vi "Autonomous Independent.vi"   [LabVIEW 2017]
doc: "This VI is called when autonomous begins, and will automatically be terminated when autonomous ends. You can carry out timed or sensor driven robot movement independently without needing to return to the caller."
uses:
  <vilib>/Rock Robotics/WPI/Utilities/WPI_GetSetVariantRefNum.vi
  <vilib>/Rock Robotics/Network Tables/NT Read String.vi
  <vilib>/Rock Robotics/Network Tables/NT Write Numeric Array.vi
  <vilib>/Rock Robotics/WPI/RobotDrive/WPI_RobotDriveArcadeDrive_Standard(NoSaturation).vi
panel:
  # "Be sure to right-click and choose Data Operations>>Make Current Value default if you want to save the array values with the VI"
types:
  T1 = typedef "WPI_JoystickDevRef.ctl" = cluster{"Device":T2}
  T2 = typedef "WPI_JoystickDeviceEnum.ctl" = enum16{"USB 0", "USB 1", "USB 2", "USB 3", "USB 4", "USB 5"}
  T3 = typedef "WPI_RobotDriveDevRef.ctl" = cluster{"DevStatus":errorcluster, "Motors[]":T4[], "Square Inputs":bool, "Max Output":dbl}
  T4 = typedef "WPI_MotorControlDeviceRef.ctl" = cluster{"DeviceStatus":errorcluster, "Type":T5, "PWM":cluster{"PWM Channel":T6, "DeadBand":T7}, "CAN":cluster{"Device Number":u8, "SetOutput VI Ref":variant, "GetOutput VI Ref":variant, "Enable VI Ref":variant, "Disable VI Ref":variant, "Data":variant}, "Invert":bool, "DIO PWM":cluster{"PWM \"Enable\" Channel":T6, "DIOChannel":T8, "PWM Rate":dbl}}
  T5 = typedef "WPI_MotorControlType.ctl" = enum16{"PWM", "CAN", "DIO PWM"}
  T6 = typedef "FPGA_DIOPWMChannel.ctl" = enum8{"PWM 0", "PWM 1", "PWM 2", "PWM 3", "PWM 4", "PWM 5", "PWM 6", "PWM 7", "PWM 8", "PWM 9", "PWM MXP 0", "PWM MXP 1", "PWM MXP 2", "PWM MXP 3", "PWM MXP 4", "PWM MXP 5", "PWM MXP 6", "PWM MXP 7", "PWM MXP 8", "PWM MXP 9", "Invalid"}
  T7 = typedef "WPI_PWMDeadband.ctl" = cluster{"Name":string, "maxPositivePwm":i32, "minPositivePwm":i32, "centerPwm":i32, "maxNegativePwm":i32, "minNegativePwm":i32, "angularRange":u16}
  T8 = typedef "FPGA_DIOChannel.ctl" = enum8{"DIO 0", "DIO 1", "DIO 2", "DIO 3", "DIO 4", "DIO 5", "DIO 6", "DIO 7", "DIO 8", "DIO 9", "DIO MXP 0", "DIO MXP 1", "DIO MXP 2", "DIO MXP 3", "DIO MXP 4", "DIO MXP 5", "DIO MXP 6", "DIO MXP 7", "DIO MXP 8", "DIO MXP 9", "DIO MXP 10", "DIO MXP 11", "DIO MXP 12", "DIO MXP 13", "DIO MXP 14", "DIO MXP 15", "SPI Port CS1", "SPI Port CS2", "SPI Port CS3", "SPI Port MISO", "SPI Port MOSI", "Invalid"}
  T9 = typedef "WPI_SwitchDevRef.ctl" = cluster{"DevStatus":errorcluster, "DIO Channel":T8, "CntIndex":T10, "Normally Closed":bool}
  T10 = typedef "FPGA_CounterCtrSystemIndex.ctl" = enum8{"Ctr 0", "Ctr 1", "Ctr 2", "Ctr 3", "Ctr 4", "Ctr 5", "Ctr 6", "Ctr 7", "Invalid"}
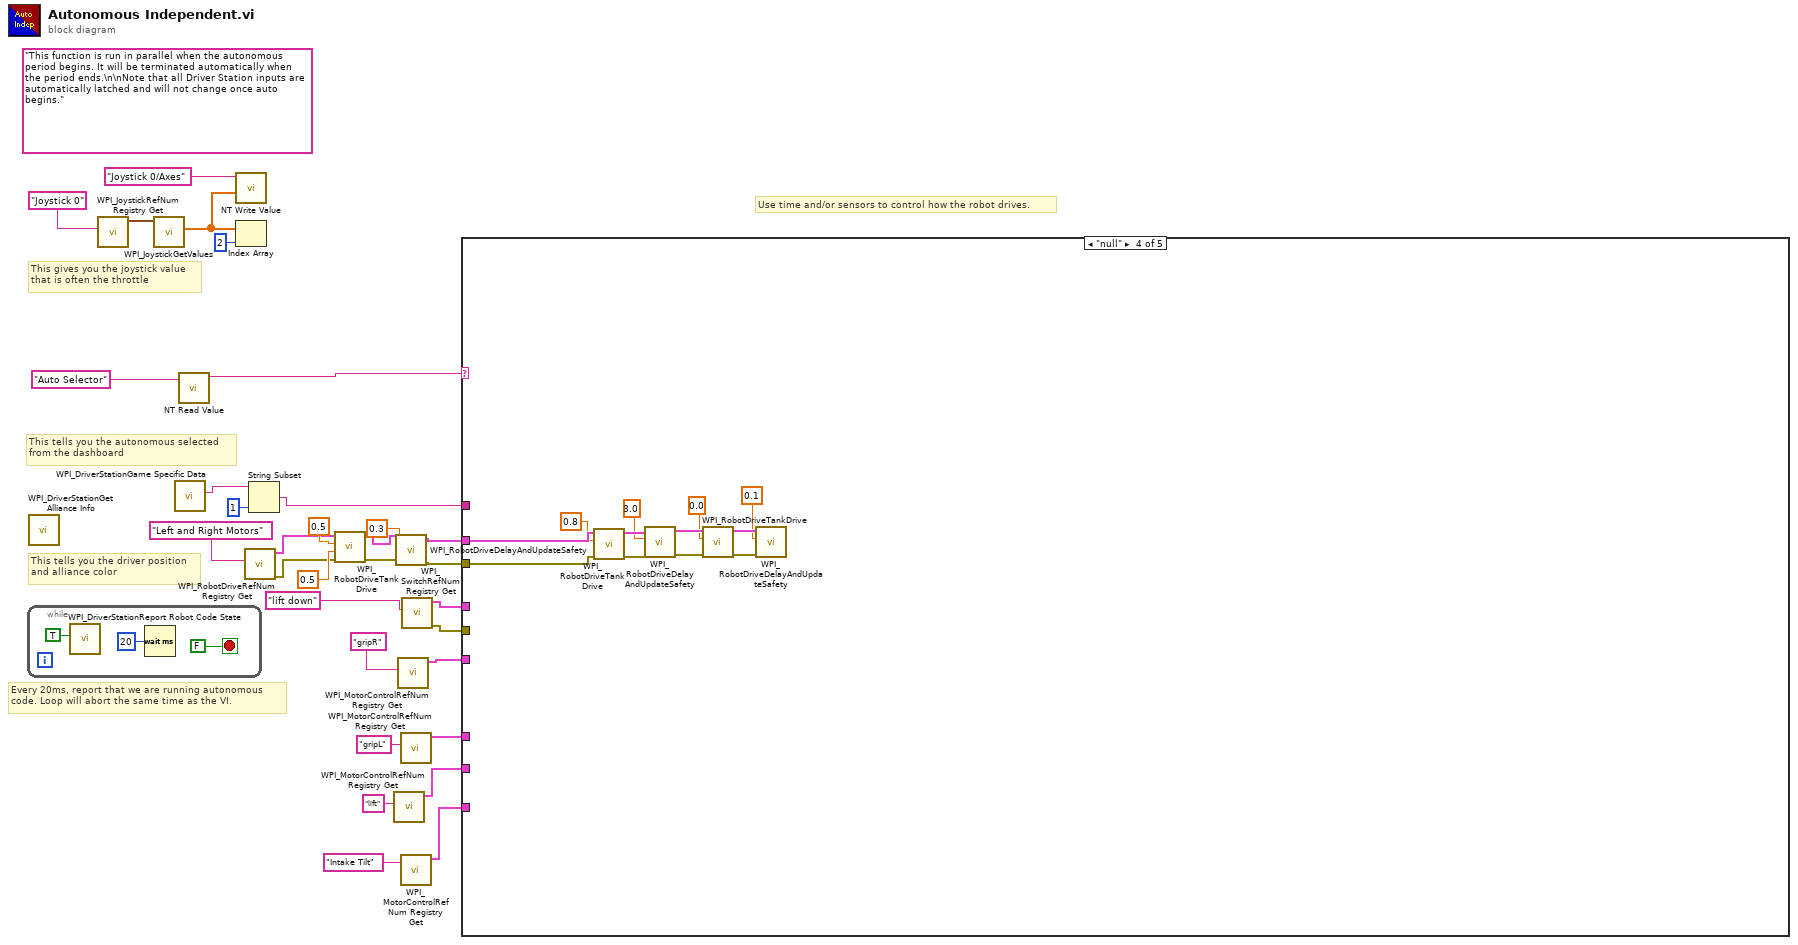
[diagram p0: block diagram]
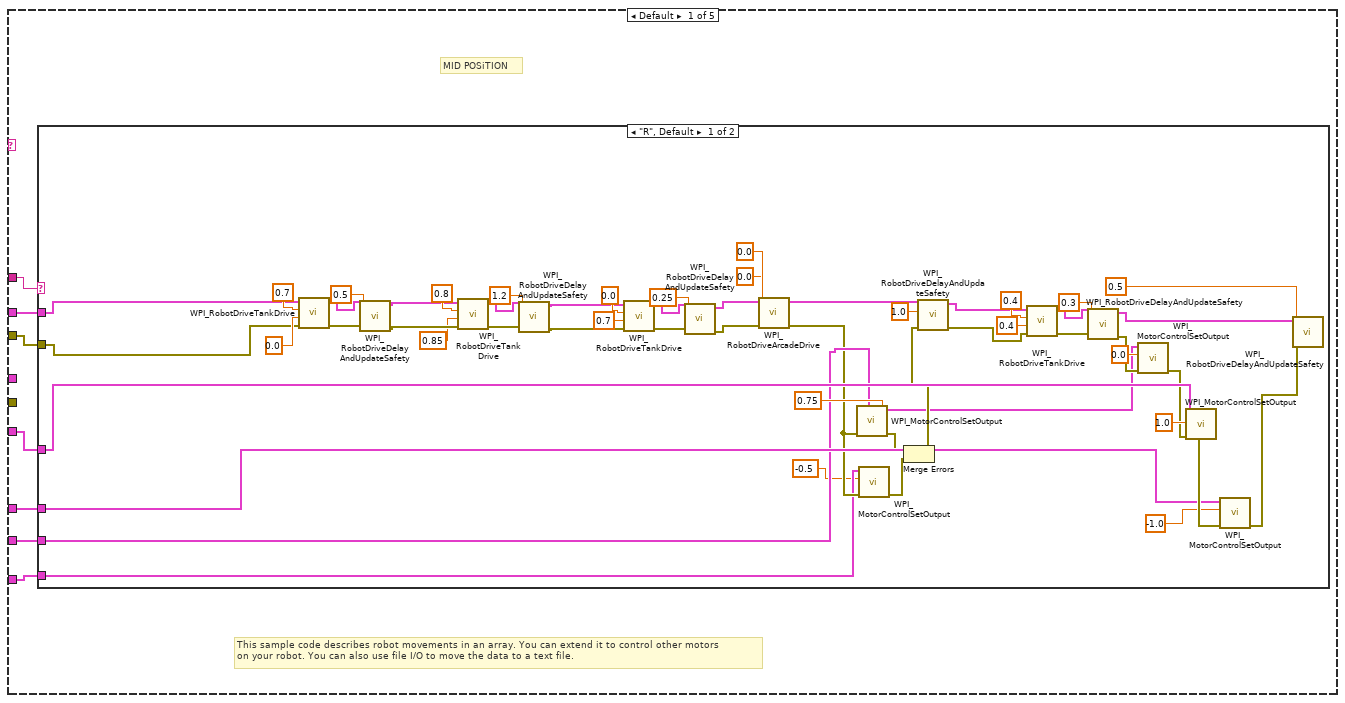
[diagram p2: hidden frame]
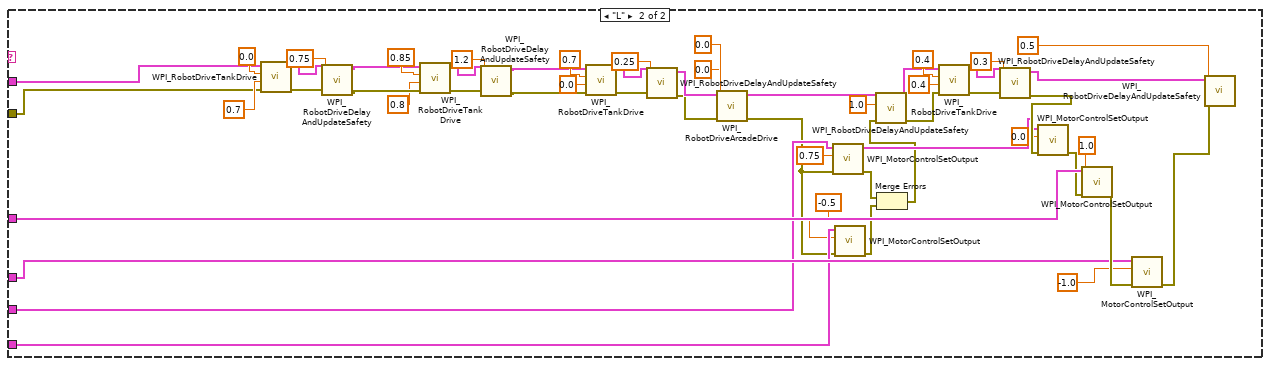
[diagram p3: hidden frame]
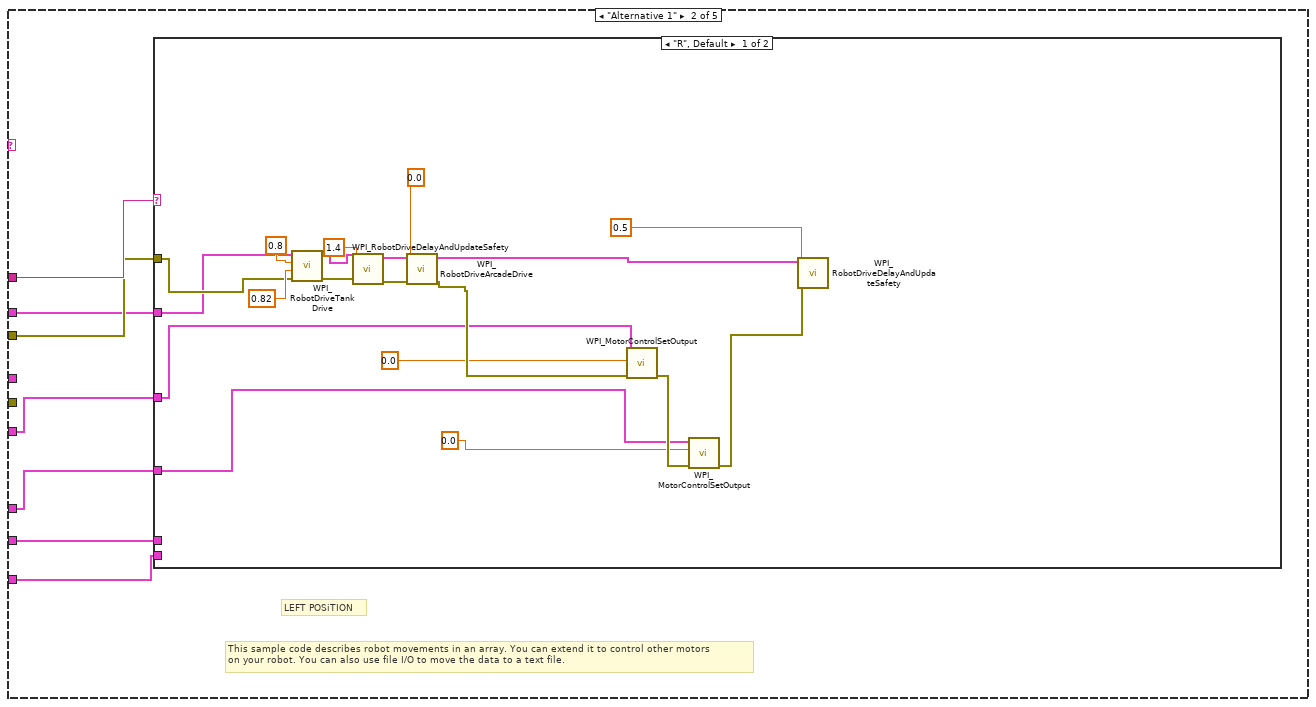
[diagram p4: hidden frame]
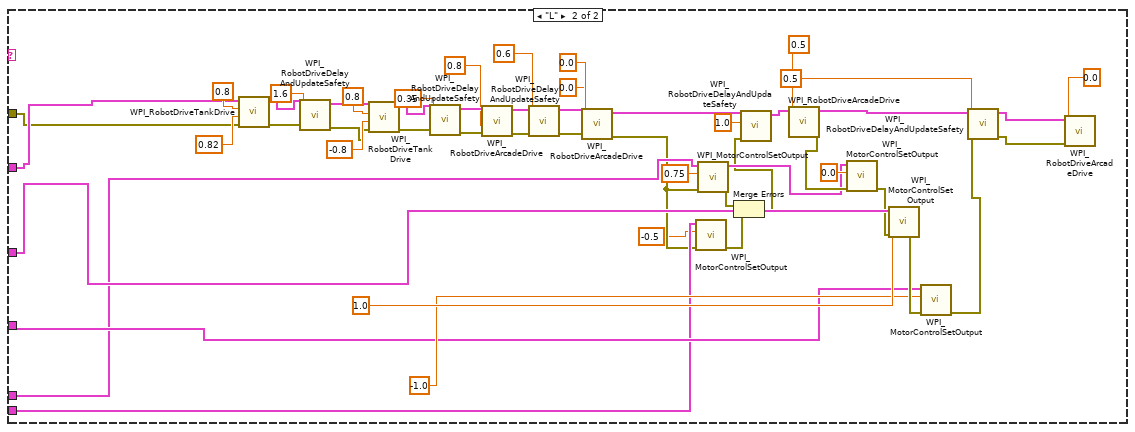
[diagram p5: hidden frame]
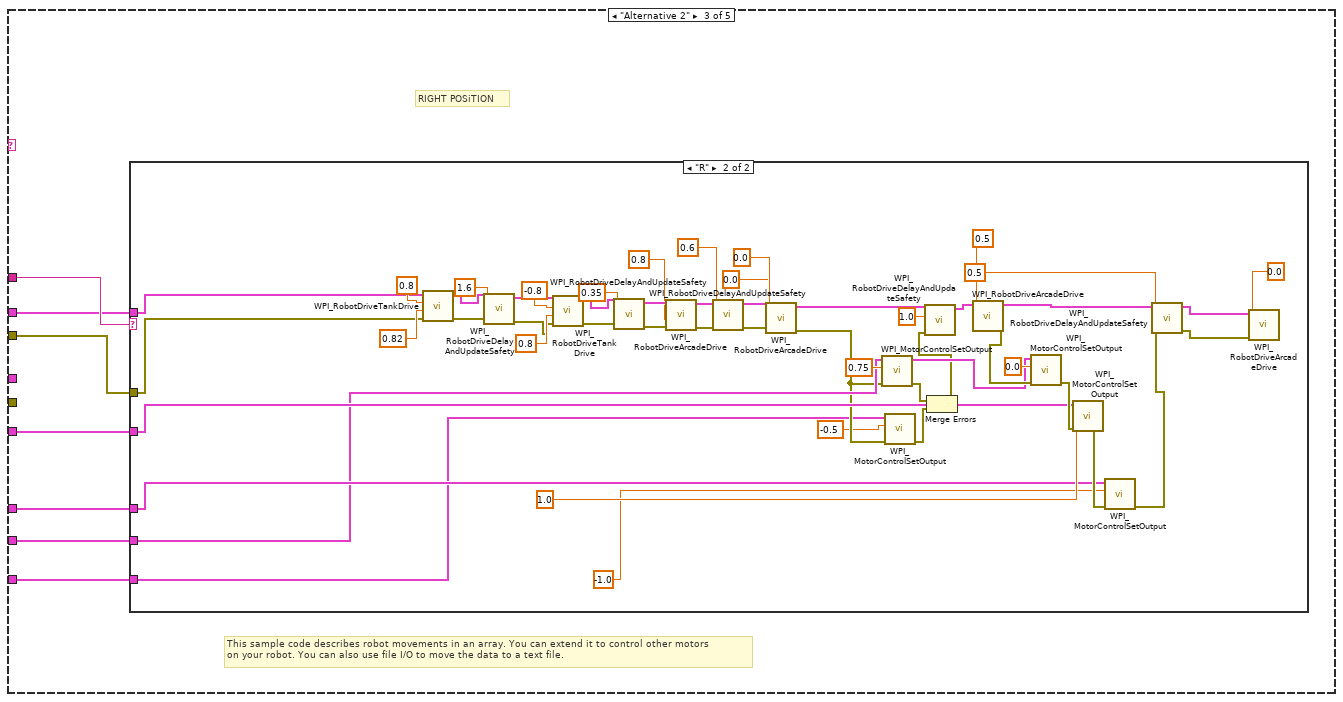
[diagram p6: hidden frame]
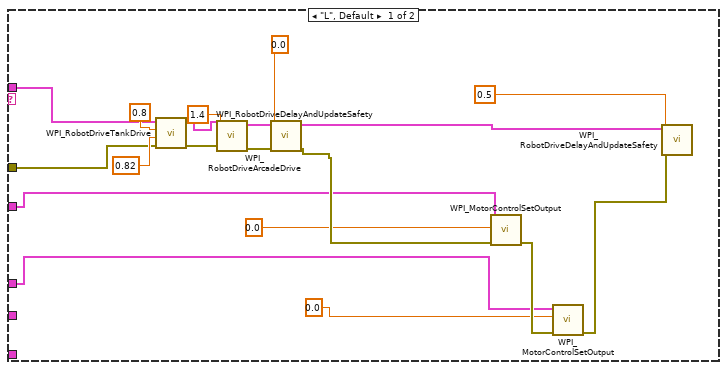
[diagram p7: hidden frame]
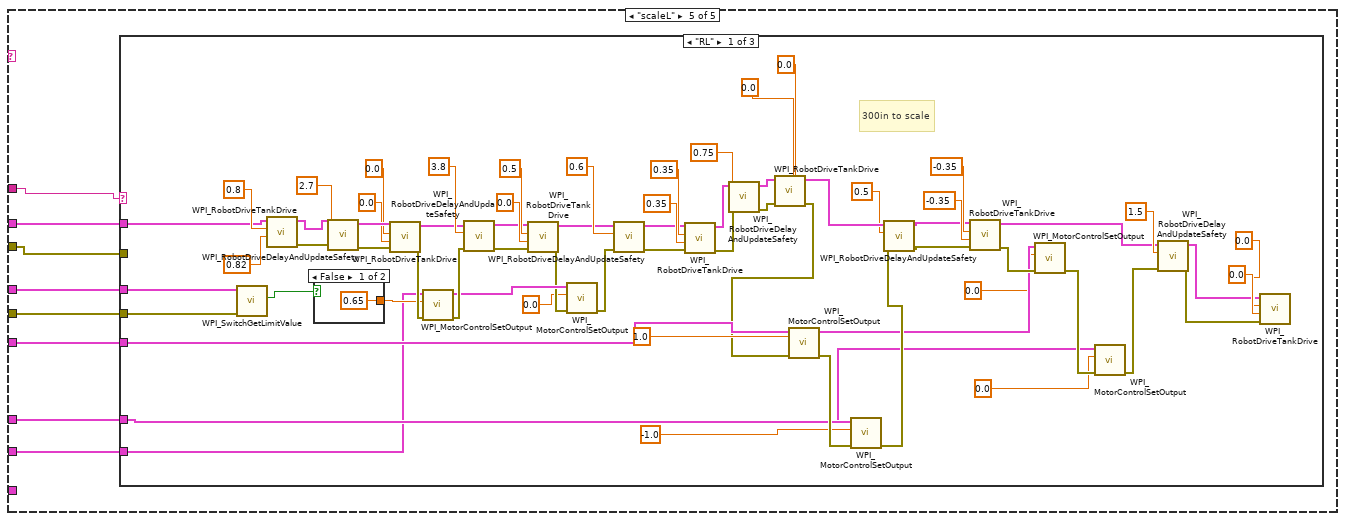
[diagram p8: hidden frame]
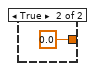
[diagram p9: hidden frame]
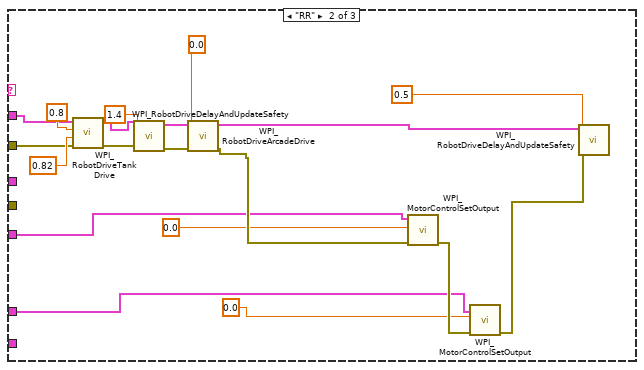
[diagram p10: hidden frame]
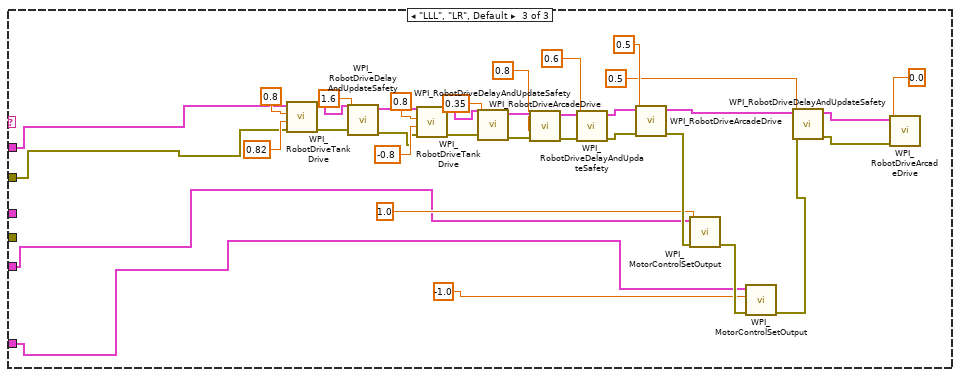
[diagram p11: hidden frame]
diagram:
  (unwired) "This function is run in parallel when the autonomous period begins. It will be terminated automatically when the period ends.\n\nNote that all Driver Station inputs are automatically latched and will not change once auto begins."
  # "This tells you the autonomous selected\nfrom the dashboard"
  # "Every 20ms, report that we are running autonomous\ncode. Loop will abort the same time as the VI."
  # "This gives you the joystick value\nthat is often the throttle"
  # "Use time and/or sensors to control how the robot drives."
  # "This tells you the driver position\nand alliance color"
  n1 = while {
    stop <- FALSE stop-if-true
    n2 = call <vilib>:"WPI_DriverStationReport Robot Code State.vi"("Autonomous"=TRUE) -> ()  [unwired: 10 in, 1 out]
    n3 = Wait (ms)(milliseconds to wait=u32 20) -> ()  [unwired: 1 out]
  }
  n4 = call <vilib>:"WPI_DriverStationGet Alliance Info.vi"() -> ()  [unwired: 12 out]
  n5 = call <vilib>:"WPI_JoystickRefNum Registry Get.vi"("refnum name"="Joystick 0") -> ("JoystickDevRef"=w30:T1)  [unwired: 1 in, 9 out]
  n6 = call <vilib>:"WPI_JoystickGetValues.vi"("JoystickDevRef"=w30) -> ("Axes"=w26:dbl[])  [unwired: 6 in, 4 out]
  n7 = call <vilib>:"WPI_DriverStationGame Specific Data.vi"() -> ("Game Specific Data"=w24:string)  [unwired: 11 in]
  n8 = call-poly <vilib>:"NT Read Value.vi"("Name"="Auto Selector") -> ("String"=w27:string)  [unwired: 9 in, 1 out]
  n9 = call-poly <vilib>:"NT Write Value.vi"("Numeric Array"=w26, "Name"="Joystick 0/Axes") -> ()  [unwired: 9 in, 1 out]
  n10 = Index Array(array=w26, index=2) -> ()  [unwired: 1 out]
  n11 = call <vilib>:"WPI_RobotDriveRefNum Registry Get.vi"("refnum name"="Left and Right Motors") -> ("error out"=w6:errorcluster, "RobotDriveDevRef"=w5:T3)  [unwired: 1 in, 8 out]
  n12 = String Subset(string=w24, length (rest)=1 ("length (rest)")) -> (substring=w22:string)  [unwired: 1 in]
  n13 = call <vilib>:"WPI_RobotDriveTankDrive.vi"("error in (no error)"=w6, "Right axis value"=0.5 ("Y axis value"), "Left axis value"=0.5 ("X axis value"), "RobotDriveDevRef"=w5) -> ("error out"=w10:errorcluster, "RobotDriveDevRef"=w9:T3)  [unwired: 5 in, 1 out]
  n14 = call <vilib>:"WPI_MotorControlRefNum Registry Get.vi"("refnum name"="lift") -> ("MotorControlDevRef"=w12:T4)  [unwired: 9 in, 1 out]
  n15 = call <vilib>:"WPI_RobotDriveDelayAndUpdateSafety.vi"("error in (no error)"=w10, "Delay (s)"=0.3, "RobotDriveDevRef"=w9) -> ("error out"=w3:errorcluster, "RobotDriveDevRef 2"=w4:T3)  [unwired: 7 in]
  n16 = call <vilib>:"WPI_MotorControlRefNum Registry Get.vi"("refnum name"="gripR") -> ("MotorControlDevRef"=w19:T4)  [unwired: 9 in, 1 out]
  n17 = call <vilib>:"WPI_MotorControlRefNum Registry Get.vi"("refnum name"="gripL") -> ("MotorControlDevRef"=w17:T4)  [unwired: 9 in, 1 out]
  n18 = call <vilib>:"WPI_MotorControlRefNum Registry Get.vi"("refnum name"="Intake Tilt") -> ("MotorControlDevRef"=w2:T4)  [unwired: 9 in, 1 out]
  n19 = call <vilib>:"WPI_SwitchRefNum Registry Get.vi"("refnum name"="lift down") -> ("error out"=w14:errorcluster, "SwitchDevRef"=w13:T9)  [unwired: 9 in]
  n20 = case shown="\"null\"" w27 {
    tunnel: w22 -> [w41 w156 w233 _ w323]
    tunnel: w3 -> [w40 w155 w232 w312 w316]
    tunnel: w19 -> [w39 w154 w231 _ w320]
    tunnel: w17 -> [w38 w153 w230 _ w321]
    tunnel: w4 -> [w37 w152 w229 w313 w322]
    tunnel: w14 -> [_ _ _ _ w319]
    tunnel: w13 -> [_ _ _ _ w318]
    tunnel: w12 -> [w36 w151 w228 _ w317]
    tunnel: w2 -> [w35 w150 w227 _ _]
    frame Default {
      # "MID POSiTION"
      # "This sample code describes robot movements in an array. You can extend it to control other motors\non your robot. You can also use file I/O to move the data to a text file."
      n21 = case shown="\"R\", Default" w41 {
        tunnel: w40 -> [w85 w119]
        tunnel: w39 -> [w84 w118]
        tunnel: w38 -> [w83 w117]
        tunnel: w37 -> [w62 w116]
        tunnel: w36 -> [w52 w106]
        tunnel: w35 -> [w44 w101]
        frame "R", Default {
          n22 = call <vilib>:"WPI_RobotDriveTankDrive.vi"("error in (no error)"=w85, "Right axis value"=0.0 ("Y axis value"), "Left axis value"=0.7 ("X axis value"), "RobotDriveDevRef"=w62) -> ("error out"=w91:errorcluster, "RobotDriveDevRef"=w90:T3)  [unwired: 5 in, 1 out]
          n23 = call <vilib>:"WPI_RobotDriveDelayAndUpdateSafety.vi"("error in (no error)"=w91, "Delay (s)"=0.5, "RobotDriveDevRef"=w90) -> ("error out"=w77:errorcluster, "RobotDriveDevRef 2"=w78:T3)  [unwired: 7 in]
          n24 = call <vilib>:"WPI_RobotDriveTankDrive.vi"("error in (no error)"=w77, "Right axis value"=0.85, "Left axis value"=0.8 ("X axis value"), "RobotDriveDevRef"=w78) -> ("error out"=w81:errorcluster, "RobotDriveDevRef"=w80:T3)  [unwired: 5 in, 1 out]
          n25 = call <vilib>:"WPI_RobotDriveDelayAndUpdateSafety.vi"("error in (no error)"=w81, "Delay (s)"=1.2, "RobotDriveDevRef"=w80) -> ("error out"=w70:errorcluster, "RobotDriveDevRef 2"=w71:T3)  [unwired: 7 in]
          n26 = call <vilib>:"WPI_RobotDriveTankDrive.vi"("error in (no error)"=w70, "Right axis value"=0.7, "Left axis value"=0.0 ("X axis value"), "RobotDriveDevRef"=w71) -> ("error out"=w74:errorcluster, "RobotDriveDevRef"=w73:T3)  [unwired: 5 in, 1 out]
          n27 = call <vilib>:"WPI_RobotDriveDelayAndUpdateSafety.vi"("error in (no error)"=w74, "Delay (s)"=0.25, "RobotDriveDevRef"=w73) -> ("error out"=w55:errorcluster, "RobotDriveDevRef 2"=w56:T3)  [unwired: 7 in]
          n28 = call-poly <vilib>:"WPI_RobotDriveArcadeDrive.vi"("error in (no error)"=w55, "Y axis value"=0.0, "X axis value"=0.0, "RobotDriveDevRef"=w56) -> ("error out"=w48:errorcluster, "RobotDriveDevRef"=w61:T3)  [unwired: 5 in, 1 out]
          n29 = call <vilib>:"WPI_MotorControlSetOutput.vi"("error in (no error)"=w48, "Output"=0.75, "MotorControlDevRef"=w52) -> ("error out"=w47:errorcluster, "MotorControlDevRef"=w42:T4)  [unwired: 6 in, 1 out]
          n30 = call <vilib>:"WPI_MotorControlSetOutput.vi"("error in (no error)"=w48, "Output"=-0.5, "MotorControlDevRef"=w44) -> ("error out"=w46:errorcluster)  [unwired: 6 in, 2 out]
          n31 = Merge Errors(w47, w46) -> (w45:errorcluster)
          n32 = call <vilib>:"WPI_RobotDriveDelayAndUpdateSafety.vi"("error in (no error)"=w45, "Delay (s)"=1.0, "RobotDriveDevRef"=w61) -> ("error out"=w53:errorcluster, "RobotDriveDevRef 2"=w54:T3)  [unwired: 7 in]
          n33 = call <vilib>:"WPI_RobotDriveTankDrive.vi"("error in (no error)"=w53, "Right axis value"=0.4, "Left axis value"=0.4 ("X axis value"), "RobotDriveDevRef"=w54) -> ("error out"=w67:errorcluster, "RobotDriveDevRef"=w66:T3)  [unwired: 5 in, 1 out]
          n34 = call <vilib>:"WPI_RobotDriveDelayAndUpdateSafety.vi"("error in (no error)"=w67, "Delay (s)"=0.3, "RobotDriveDevRef"=w66) -> ("error out"=w51:errorcluster, "RobotDriveDevRef 2"=w63:T3)  [unwired: 7 in]
          n35 = call <vilib>:"WPI_MotorControlSetOutput.vi"("error in (no error)"=w51, "Output"=0.0, "MotorControlDevRef"=w42) -> ("error out"=w50:errorcluster)  [unwired: 6 in, 2 out]
          n36 = call <vilib>:"WPI_MotorControlSetOutput.vi"("error in (no error)"=w50, "Output"=1.0, "MotorControlDevRef"=w84) -> ("error out"=w93:errorcluster)  [unwired: 6 in, 2 out]
          n37 = call <vilib>:"WPI_MotorControlSetOutput.vi"("error in (no error)"=w93, "Output"=-1.0, "MotorControlDevRef"=w83) -> ("error out"=w92:errorcluster)  [unwired: 6 in, 2 out]
          n38 = call <vilib>:"WPI_RobotDriveDelayAndUpdateSafety.vi"("error in (no error)"=w92, "Delay (s)"=0.5, "RobotDriveDevRef"=w63) -> ()  [unwired: 7 in, 2 out]
        }
        frame "L" {
          n39 = call <vilib>:"WPI_RobotDriveTankDrive.vi"("error in (no error)"=w119, "Right axis value"=0.7 ("Y axis value"), "Left axis value"=0.0 ("X axis value"), "RobotDriveDevRef"=w116) -> ("error out"=w145:errorcluster, "RobotDriveDevRef"=w144:T3)  [unwired: 5 in, 1 out]
          n40 = call <vilib>:"WPI_RobotDriveDelayAndUpdateSafety.vi"("error in (no error)"=w145, "Delay (s)"=0.75, "RobotDriveDevRef"=w144) -> ("error out"=w134:errorcluster, "RobotDriveDevRef 2"=w135:T3)  [unwired: 7 in]
          n41 = call <vilib>:"WPI_RobotDriveTankDrive.vi"("error in (no error)"=w134, "Right axis value"=0.8, "Left axis value"=0.85 ("X axis value"), "RobotDriveDevRef"=w135) -> ("error out"=w138:errorcluster, "RobotDriveDevRef"=w137:T3)  [unwired: 5 in, 1 out]
          n42 = call <vilib>:"WPI_RobotDriveDelayAndUpdateSafety.vi"("error in (no error)"=w138, "Delay (s)"=1.2, "RobotDriveDevRef"=w137) -> ("error out"=w127:errorcluster, "RobotDriveDevRef 2"=w128:T3)  [unwired: 7 in]
          n43 = call <vilib>:"WPI_RobotDriveTankDrive.vi"("error in (no error)"=w127, "Right axis value"=0.0, "Left axis value"=0.7 ("X axis value"), "RobotDriveDevRef"=w128) -> ("error out"=w131:errorcluster, "RobotDriveDevRef"=w130:T3)  [unwired: 5 in, 1 out]
          n44 = call <vilib>:"WPI_RobotDriveDelayAndUpdateSafety.vi"("error in (no error)"=w131, "Delay (s)"=0.25, "RobotDriveDevRef"=w130) -> ("error out"=w109:errorcluster, "RobotDriveDevRef 2"=w110:T3)  [unwired: 7 in]
          n45 = call-poly <vilib>:"WPI_RobotDriveArcadeDrive.vi"("error in (no error)"=w109, "Y axis value"=0.0, "X axis value"=0.0, "RobotDriveDevRef"=w110) -> ("error out"=w100:errorcluster, "RobotDriveDevRef"=w115:T3)  [unwired: 5 in, 1 out]
          n46 = call <vilib>:"WPI_MotorControlSetOutput.vi"("error in (no error)"=w100, "Output"=0.75, "MotorControlDevRef"=w106) -> ("error out"=w99:errorcluster, "MotorControlDevRef"=w103:T4)  [unwired: 6 in, 1 out]
          n47 = call <vilib>:"WPI_MotorControlSetOutput.vi"("error in (no error)"=w100, "Output"=-0.5, "MotorControlDevRef"=w101) -> ("error out"=w98:errorcluster)  [unwired: 6 in, 2 out]
          n48 = Merge Errors(w99, w98) -> (w97:errorcluster)
          n49 = call <vilib>:"WPI_RobotDriveDelayAndUpdateSafety.vi"("error in (no error)"=w97, "Delay (s)"=1.0, "RobotDriveDevRef"=w115) -> ("error out"=w107:errorcluster, "RobotDriveDevRef 2"=w108:T3)  [unwired: 7 in]
          n50 = call <vilib>:"WPI_RobotDriveTankDrive.vi"("error in (no error)"=w107, "Right axis value"=0.4, "Left axis value"=0.4 ("X axis value"), "RobotDriveDevRef"=w108) -> ("error out"=w124:errorcluster, "RobotDriveDevRef"=w123:T3)  [unwired: 5 in, 1 out]
          n51 = call <vilib>:"WPI_RobotDriveDelayAndUpdateSafety.vi"("error in (no error)"=w124, "Delay (s)"=0.3, "RobotDriveDevRef"=w123) -> ("error out"=w105:errorcluster, "RobotDriveDevRef 2"=w120:T3)  [unwired: 7 in]
          n52 = call <vilib>:"WPI_MotorControlSetOutput.vi"("error in (no error)"=w105, "Output"=0.0, "MotorControlDevRef"=w103) -> ("error out"=w104:errorcluster)  [unwired: 6 in, 2 out]
          n53 = call <vilib>:"WPI_MotorControlSetOutput.vi"("error in (no error)"=w104, "Output"=1.0, "MotorControlDevRef"=w118) -> ("error out"=w147:errorcluster)  [unwired: 6 in, 2 out]
          n54 = call <vilib>:"WPI_MotorControlSetOutput.vi"("error in (no error)"=w147, "Output"=-1.0, "MotorControlDevRef"=w117) -> ("error out"=w146:errorcluster)  [unwired: 6 in, 2 out]
          n55 = call <vilib>:"WPI_RobotDriveDelayAndUpdateSafety.vi"("error in (no error)"=w146, "Delay (s)"=0.5, "RobotDriveDevRef"=w120) -> ()  [unwired: 7 in, 2 out]
        }
      }
    }
    frame "Alternative 1" {
      # "LEFT POSiTION"
      # "This sample code describes robot movements in an array. You can extend it to control other motors\non your robot. You can also use file I/O to move the data to a text file."
      n56 = case shown="\"R\", Default" w156 {
        tunnel: w155 -> [w160 w206]
        tunnel: w154 -> [w159 w205]
        tunnel: w153 -> [w158 w204]
        tunnel: w152 -> [w157 w207]
        tunnel: w151 -> [_ w186]
        tunnel: w150 -> [_ w181]
        frame "R", Default {
          n57 = call <vilib>:"WPI_RobotDriveTankDrive.vi"("error in (no error)"=w160, "Right axis value"=0.82 ("Y axis value"), "Left axis value"=0.8 ("X axis value"), "RobotDriveDevRef"=w157) -> ("error out"=w166:errorcluster, "RobotDriveDevRef"=w165:T3)  [unwired: 5 in, 1 out]
          n58 = call <vilib>:"WPI_RobotDriveDelayAndUpdateSafety.vi"("error in (no error)"=w166, "Delay (s)"=1.4, "RobotDriveDevRef"=w165) -> ("error out"=w174:errorcluster, "RobotDriveDevRef 2"=w173:T3)  [unwired: 7 in]
          n59 = call-poly <vilib>:"WPI_RobotDriveArcadeDrive.vi"("error in (no error)"=w174, "Y axis value"=0.0, "RobotDriveDevRef"=w173) -> ("error out"=w168:errorcluster, "RobotDriveDevRef"=w171:T3)  [unwired: 6 in, 1 out]
          n60 = call <vilib>:"WPI_MotorControlSetOutput.vi"("error in (no error)"=w168, "Output"=0.0, "MotorControlDevRef"=w159) -> ("error out"=w169:errorcluster)  [unwired: 6 in, 2 out]
          n61 = call <vilib>:"WPI_MotorControlSetOutput.vi"("error in (no error)"=w169, "Output"=0.0, "MotorControlDevRef"=w158) -> ("error out"=w167:errorcluster)  [unwired: 6 in, 2 out]
          n62 = call <vilib>:"WPI_RobotDriveDelayAndUpdateSafety.vi"("error in (no error)"=w167, "Delay (s)"=0.5, "RobotDriveDevRef"=w171) -> ()  [unwired: 7 in, 2 out]
        }
        frame "L" {
          n63 = call <vilib>:"WPI_RobotDriveTankDrive.vi"("error in (no error)"=w206, "Right axis value"=0.82 ("Y axis value"), "Left axis value"=0.8 ("X axis value"), "RobotDriveDevRef"=w207) -> ("error out"=w220:errorcluster, "RobotDriveDevRef"=w219:T3)  [unwired: 5 in, 1 out]
          n64 = call <vilib>:"WPI_RobotDriveDelayAndUpdateSafety.vi"("error in (no error)"=w220, "Delay (s)"=1.6, "RobotDriveDevRef"=w219) -> ("error out"=w208:errorcluster, "RobotDriveDevRef 2"=w209:T3)  [unwired: 7 in]
          n65 = call <vilib>:"WPI_RobotDriveTankDrive.vi"("error in (no error)"=w208, "Right axis value"=-0.8 ("Y axis value"), "Left axis value"=0.8 ("X axis value"), "RobotDriveDevRef"=w209) -> ("error out"=w213:errorcluster, "RobotDriveDevRef"=w212:T3)  [unwired: 5 in, 1 out]
          n66 = call <vilib>:"WPI_RobotDriveDelayAndUpdateSafety.vi"("error in (no error)"=w213, "Delay (s)"=0.35, "RobotDriveDevRef"=w212) -> ("error out"=w199:errorcluster, "RobotDriveDevRef 2"=w200:T3)  [unwired: 7 in]
          n67 = call-poly <vilib>:"WPI_RobotDriveArcadeDrive.vi"("error in (no error)"=w199, "Y axis value"=0.8, "RobotDriveDevRef"=w200) -> ("error out"=w196:errorcluster, "RobotDriveDevRef"=w197:T3)  [unwired: 6 in, 1 out]
          n68 = call <vilib>:"WPI_RobotDriveDelayAndUpdateSafety.vi"("error in (no error)"=w196, "Delay (s)"=0.6, "RobotDriveDevRef"=w197) -> ("error out"=w194:errorcluster, "RobotDriveDevRef 2"=w193:T3)  [unwired: 7 in]
          n69 = call-poly <vilib>:"WPI_RobotDriveArcadeDrive.vi"("error in (no error)"=w194, "Y axis value"=0.0, "X axis value"=0.0, "RobotDriveDevRef"=w193) -> ("error out"=w180:errorcluster, "RobotDriveDevRef"=w192:T3)  [unwired: 5 in, 1 out]
          n70 = call <vilib>:"WPI_MotorControlSetOutput.vi"("error in (no error)"=w180, "Output"=-0.5, "MotorControlDevRef"=w181) -> ("error out"=w178:errorcluster)  [unwired: 6 in, 2 out]
          n71 = call <vilib>:"WPI_MotorControlSetOutput.vi"("error in (no error)"=w180, "Output"=0.75, "MotorControlDevRef"=w186) -> ("error out"=w179:errorcluster, "MotorControlDevRef"=w182:T4)  [unwired: 6 in, 1 out]
          n72 = Merge Errors(w179, w178) -> (w177:errorcluster)
          n73 = call <vilib>:"WPI_RobotDriveDelayAndUpdateSafety.vi"("error in (no error)"=w177, "Delay (s)"=1.0, "RobotDriveDevRef"=w192) -> ("RobotDriveDevRef 2"=w191:T3)  [unwired: 7 in, 1 out]
          n74 = call-poly <vilib>:"WPI_RobotDriveArcadeDrive.vi"("Y axis value"=0.5, "RobotDriveDevRef"=w191) -> ("error out"=w184:errorcluster, "RobotDriveDevRef"=w224:T3)  [unwired: 7 in, 1 out]
          n75 = call <vilib>:"WPI_MotorControlSetOutput.vi"("error in (no error)"=w184, "Output"=0.0, "MotorControlDevRef"=w182) -> ("error out"=w183:errorcluster)  [unwired: 6 in, 2 out]
          n76 = call <vilib>:"WPI_MotorControlSetOutput.vi"("error in (no error)"=w183, "Output"=1.0, "MotorControlDevRef"=w205) -> ("error out"=w222:errorcluster)  [unwired: 6 in, 2 out]
          n77 = call <vilib>:"WPI_MotorControlSetOutput.vi"("error in (no error)"=w222, "Output"=-1.0, "MotorControlDevRef"=w204) -> ("error out"=w221:errorcluster)  [unwired: 6 in, 2 out]
          n78 = call <vilib>:"WPI_RobotDriveDelayAndUpdateSafety.vi"("error in (no error)"=w221, "Delay (s)"=0.5, "RobotDriveDevRef"=w224) -> ("error out"=w201:errorcluster, "RobotDriveDevRef 2"=w202:T3)  [unwired: 7 in]
          n79 = call-poly <vilib>:"WPI_RobotDriveArcadeDrive.vi"("error in (no error)"=w201, "Y axis value"=0.0, "RobotDriveDevRef"=w202) -> ()  [unwired: 6 in, 3 out]
        }
      }
    }
    frame "Alternative 2" {
      # "RIGHT POSiTION"
      # "This sample code describes robot movements in an array. You can extend it to control other motors\non your robot. You can also use file I/O to move the data to a text file."
      n80 = case shown="\"R\"" w233 {
        tunnel: w232 -> [w235 w262]
        tunnel: w231 -> [w236 w261]
        tunnel: w230 -> [w237 w260]
        tunnel: w229 -> [w234 w263]
        tunnel: w228 -> [_ w259]
        tunnel: w227 -> [_ w257]
        frame "L", Default {
          n81 = call <vilib>:"WPI_RobotDriveTankDrive.vi"("error in (no error)"=w235, "Right axis value"=0.82 ("Y axis value"), "Left axis value"=0.8 ("X axis value"), "RobotDriveDevRef"=w234) -> ("error out"=w243:errorcluster, "RobotDriveDevRef"=w242:T3)  [unwired: 5 in, 1 out]
          n82 = call <vilib>:"WPI_RobotDriveDelayAndUpdateSafety.vi"("error in (no error)"=w243, "Delay (s)"=1.4, "RobotDriveDevRef"=w242) -> ("error out"=w251:errorcluster, "RobotDriveDevRef 2"=w250:T3)  [unwired: 7 in]
          n83 = call-poly <vilib>:"WPI_RobotDriveArcadeDrive.vi"("error in (no error)"=w251, "Y axis value"=0.0, "RobotDriveDevRef"=w250) -> ("error out"=w245:errorcluster, "RobotDriveDevRef"=w248:T3)  [unwired: 6 in, 1 out]
          n84 = call <vilib>:"WPI_MotorControlSetOutput.vi"("error in (no error)"=w245, "Output"=0.0, "MotorControlDevRef"=w236) -> ("error out"=w246:errorcluster)  [unwired: 6 in, 2 out]
          n85 = call <vilib>:"WPI_MotorControlSetOutput.vi"("error in (no error)"=w246, "Output"=0.0, "MotorControlDevRef"=w237) -> ("error out"=w244:errorcluster)  [unwired: 6 in, 2 out]
          n86 = call <vilib>:"WPI_RobotDriveDelayAndUpdateSafety.vi"("error in (no error)"=w244, "Delay (s)"=0.5, "RobotDriveDevRef"=w248) -> ()  [unwired: 7 in, 2 out]
        }
        frame "R" {
          n87 = call <vilib>:"WPI_RobotDriveTankDrive.vi"("error in (no error)"=w262, "Right axis value"=0.82 ("Y axis value"), "Left axis value"=0.8 ("X axis value"), "RobotDriveDevRef"=w263) -> ("error out"=w297:errorcluster, "RobotDriveDevRef"=w296:T3)  [unwired: 5 in, 1 out]
          n88 = call <vilib>:"WPI_RobotDriveDelayAndUpdateSafety.vi"("error in (no error)"=w297, "Delay (s)"=1.6, "RobotDriveDevRef"=w296) -> ("error out"=w285:errorcluster, "RobotDriveDevRef 2"=w286:T3)  [unwired: 7 in]
          n89 = call <vilib>:"WPI_RobotDriveTankDrive.vi"("error in (no error)"=w285, "Right axis value"=0.8 ("Y axis value"), "Left axis value"=-0.8 ("X axis value"), "RobotDriveDevRef"=w286) -> ("error out"=w290:errorcluster, "RobotDriveDevRef"=w289:T3)  [unwired: 5 in, 1 out]
          n90 = call <vilib>:"WPI_RobotDriveDelayAndUpdateSafety.vi"("error in (no error)"=w290, "Delay (s)"=0.35, "RobotDriveDevRef"=w289) -> ("error out"=w280:errorcluster, "RobotDriveDevRef 2"=w281:T3)  [unwired: 7 in]
          n91 = call-poly <vilib>:"WPI_RobotDriveArcadeDrive.vi"("error in (no error)"=w280, "Y axis value"=0.8, "RobotDriveDevRef"=w281) -> ("error out"=w277:errorcluster, "RobotDriveDevRef"=w278:T3)  [unwired: 6 in, 1 out]
          n92 = call <vilib>:"WPI_RobotDriveDelayAndUpdateSafety.vi"("error in (no error)"=w277, "Delay (s)"=0.6, "RobotDriveDevRef"=w278) -> ("error out"=w275:errorcluster, "RobotDriveDevRef 2"=w274:T3)  [unwired: 7 in]
          n93 = call-poly <vilib>:"WPI_RobotDriveArcadeDrive.vi"("error in (no error)"=w275, "Y axis value"=0.0, "X axis value"=0.0, "RobotDriveDevRef"=w274) -> ("error out"=w258:errorcluster, "RobotDriveDevRef"=w273:T3)  [unwired: 5 in, 1 out]
          n94 = call <vilib>:"WPI_MotorControlSetOutput.vi"("error in (no error)"=w258, "Output"=0.75, "MotorControlDevRef"=w259) -> ("error out"=w256:errorcluster, "MotorControlDevRef"=w264:T4)  [unwired: 6 in, 1 out]
          n95 = call <vilib>:"WPI_MotorControlSetOutput.vi"("error in (no error)"=w258, "Output"=-0.5, "MotorControlDevRef"=w257) -> ("error out"=w255:errorcluster)  [unwired: 6 in, 2 out]
          n96 = Merge Errors(w256, w255) -> (w254:errorcluster)
          n97 = call <vilib>:"WPI_RobotDriveDelayAndUpdateSafety.vi"("error in (no error)"=w254, "Delay (s)"=1.0, "RobotDriveDevRef"=w273) -> ("RobotDriveDevRef 2"=w272:T3)  [unwired: 7 in, 1 out]
          n98 = call-poly <vilib>:"WPI_RobotDriveArcadeDrive.vi"("Y axis value"=0.5, "RobotDriveDevRef"=w272) -> ("error out"=w266:errorcluster, "RobotDriveDevRef"=w301:T3)  [unwired: 7 in, 1 out]
          n99 = call <vilib>:"WPI_MotorControlSetOutput.vi"("error in (no error)"=w266, "Output"=0.0, "MotorControlDevRef"=w264) -> ("error out"=w265:errorcluster)  [unwired: 6 in, 2 out]
          n100 = call <vilib>:"WPI_MotorControlSetOutput.vi"("error in (no error)"=w265, "Output"=1.0, "MotorControlDevRef"=w261) -> ("error out"=w299:errorcluster)  [unwired: 6 in, 2 out]
          n101 = call <vilib>:"WPI_MotorControlSetOutput.vi"("error in (no error)"=w299, "Output"=-1.0, "MotorControlDevRef"=w260) -> ("error out"=w298:errorcluster)  [unwired: 6 in, 2 out]
          n102 = call <vilib>:"WPI_RobotDriveDelayAndUpdateSafety.vi"("error in (no error)"=w298, "Delay (s)"=0.5, "RobotDriveDevRef"=w301) -> ("error out"=w282:errorcluster, "RobotDriveDevRef 2"=w283:T3)  [unwired: 7 in]
          n103 = call-poly <vilib>:"WPI_RobotDriveArcadeDrive.vi"("error in (no error)"=w282, "Y axis value"=0.0, "RobotDriveDevRef"=w283) -> ()  [unwired: 6 in, 3 out]
        }
      }
    }
    frame "null" {
      n104 = call <vilib>:"WPI_RobotDriveTankDrive.vi"("error in (no error)"=w312, "Left axis value"=0.8 ("Output"), "RobotDriveDevRef"=w313) -> ("error out"=w315:errorcluster, "RobotDriveDevRef"=w314:T3)  [unwired: 6 in, 1 out]
      n105 = call <vilib>:"WPI_RobotDriveDelayAndUpdateSafety.vi"("error in (no error)"=w315, "Delay (s)"=3.0 ("Output"), "RobotDriveDevRef"=w314) -> ("error out"=w311:errorcluster, "RobotDriveDevRef 2"=w310:T3)  [unwired: 7 in]
      n106 = call <vilib>:"WPI_RobotDriveTankDrive.vi"("error in (no error)"=w311, "Left axis value"=0.0 ("Output"), "RobotDriveDevRef"=w310) -> ("error out"=w309:errorcluster, "RobotDriveDevRef"=w308:T3)  [unwired: 6 in, 1 out]
      n107 = call <vilib>:"WPI_RobotDriveDelayAndUpdateSafety.vi"("error in (no error)"=w309, "Delay (s)"=0.1 ("Output"), "RobotDriveDevRef"=w308) -> ()  [unwired: 7 in, 2 out]
    }
    frame "scaleL" {
      n108 = case shown="\"RL\"" w323 {
        tunnel: w322 -> [w380 w394 w414]
        tunnel: w321 -> [w360 w392 w411]
        tunnel: w320 -> [w361 w393 w412]
        tunnel: w319 -> [w357 _ _]
        tunnel: w318 -> [w356 _ _]
        tunnel: w317 -> [w355 _ _]
        tunnel: w316 -> [_ w395 w413]
        frame "RL" {
          # "300in to scale"
          n109 = call <vilib>:"WPI_SwitchGetLimitValue.vi"("error in (no error)"=w357, "SwitchDevRef"=w356) -> ("Switch Pressed"=w358:bool)  [unwired: 7 in, 2 out]
          n110 = call <vilib>:"WPI_RobotDriveTankDrive.vi"("Right axis value"=0.82 ("Y axis value"), "Left axis value"=0.8 ("X axis value"), "RobotDriveDevRef"=w380) -> ("error out"=w386:errorcluster, "RobotDriveDevRef"=w385:T3)  [unwired: 6 in, 1 out]
          n111 = case shown="False" w358 {
            tunnel: [0.65 ("Output") 0.0 ("Output")] -> w359
            frame False {
            }
            frame True {
            }
          }
          n112 = call <vilib>:"WPI_RobotDriveDelayAndUpdateSafety.vi"("error in (no error)"=w386, "Delay (s)"=2.7, "RobotDriveDevRef"=w385) -> ("error out"=w378:errorcluster, "RobotDriveDevRef 2"=w379:T3)  [unwired: 7 in]
          n113 = call <vilib>:"WPI_RobotDriveTankDrive.vi"("error in (no error)"=w378, "Right axis value"=0.0, "Left axis value"=0.0, "RobotDriveDevRef"=w379) -> ("error out"=w375:errorcluster, "RobotDriveDevRef"=w373:T3)  [unwired: 5 in, 1 out]
          n114 = call <vilib>:"WPI_MotorControlSetOutput.vi"("error in (no error)"=w375, "Output"=w359, "MotorControlDevRef"=w355) -> ("error out"=w372:errorcluster, "MotorControlDevRef"=w354:T4)  [unwired: 6 in, 1 out]
          n115 = call <vilib>:"WPI_RobotDriveDelayAndUpdateSafety.vi"("error in (no error)"=w372, "Delay (s)"=3.8, "RobotDriveDevRef"=w373) -> ("error out"=w366:errorcluster, "RobotDriveDevRef 2"=w367:T3)  [unwired: 7 in]
          n116 = call <vilib>:"WPI_RobotDriveTankDrive.vi"("error in (no error)"=w366, "Right axis value"=0.0, "Left axis value"=0.5, "RobotDriveDevRef"=w367) -> ("error out"=w353:errorcluster, "RobotDriveDevRef"=w368:T3)  [unwired: 5 in, 1 out]
          n117 = call <vilib>:"WPI_MotorControlSetOutput.vi"("error in (no error)"=w353, "Output"=0.0, "MotorControlDevRef"=w354) -> ("error out"=w352:errorcluster)  [unwired: 6 in, 2 out]
          n118 = call <vilib>:"WPI_RobotDriveDelayAndUpdateSafety.vi"("error in (no error)"=w352, "Delay (s)"=0.6, "RobotDriveDevRef"=w368) -> ("error out"=w362:errorcluster, "RobotDriveDevRef 2"=w363:T3)  [unwired: 7 in]
          n119 = call <vilib>:"WPI_RobotDriveTankDrive.vi"("error in (no error)"=w362, "Right axis value"=0.35, "Left axis value"=0.35, "RobotDriveDevRef"=w363) -> ("error out"=w336:errorcluster, "RobotDriveDevRef"=w337:T3)  [unwired: 5 in, 1 out]
          n120 = call <vilib>:"WPI_RobotDriveDelayAndUpdateSafety.vi"("error in (no error)"=w336, "Delay (s)"=0.75, "RobotDriveDevRef"=w337) -> ("error out"=w334:errorcluster, "RobotDriveDevRef 2"=w335:T3)  [unwired: 7 in]
          n121 = call <vilib>:"WPI_RobotDriveTankDrive.vi"("error in (no error)"=w334, "Right axis value"=0.0, "Left axis value"=0.0, "RobotDriveDevRef"=w335) -> ("error out"=w333:errorcluster, "RobotDriveDevRef"=w332:T3)  [unwired: 5 in, 1 out]
          n122 = call <vilib>:"WPI_MotorControlSetOutput.vi"("error in (no error)"=w333, "Output"=1.0, "MotorControlDevRef"=w361) -> ("error out"=w388:errorcluster, "MotorControlDevRef"=w344:T4)  [unwired: 6 in, 1 out]
          n123 = call <vilib>:"WPI_MotorControlSetOutput.vi"("error in (no error)"=w388, "Output"=-1.0, "MotorControlDevRef"=w360) -> ("error out"=w387:errorcluster, "MotorControlDevRef"=w343:T4)  [unwired: 6 in, 1 out]
          n124 = call <vilib>:"WPI_RobotDriveDelayAndUpdateSafety.vi"("error in (no error)"=w387, "Delay (s)"=0.5, "RobotDriveDevRef"=w332) -> ("error out"=w347:errorcluster, "RobotDriveDevRef 2"=w348:T3)  [unwired: 7 in]
          n125 = call <vilib>:"WPI_RobotDriveTankDrive.vi"("error in (no error)"=w347, "Right axis value"=-0.35, "Left axis value"=-0.35, "RobotDriveDevRef"=w348) -> ("error out"=w345:errorcluster, "RobotDriveDevRef"=w329:T3)  [unwired: 5 in, 1 out]
          n126 = call <vilib>:"WPI_MotorControlSetOutput.vi"("error in (no error)"=w345, "Output"=0.0, "MotorControlDevRef"=w344) -> ("error out"=w346:errorcluster)  [unwired: 6 in, 2 out]
          n127 = call <vilib>:"WPI_MotorControlSetOutput.vi"("error in (no error)"=w346, "Output"=0.0, "MotorControlDevRef"=w343) -> ("error out"=w328:errorcluster)  [unwired: 6 in, 2 out]
          n128 = call <vilib>:"WPI_RobotDriveDelayAndUpdateSafety.vi"("error in (no error)"=w328, "Delay (s)"=1.5, "RobotDriveDevRef"=w329) -> ("error out"=w324:errorcluster, "RobotDriveDevRef 2"=w325:T3)  [unwired: 7 in]
          n129 = call <vilib>:"WPI_RobotDriveTankDrive.vi"("error in (no error)"=w324, "Right axis value"=0.0, "Left axis value"=0.0, "RobotDriveDevRef"=w325) -> ()  [unwired: 5 in, 3 out]
        }
        frame "RR" {
          n130 = call <vilib>:"WPI_RobotDriveTankDrive.vi"("error in (no error)"=w395, "Right axis value"=0.82 ("Y axis value"), "Left axis value"=0.8 ("X axis value"), "RobotDriveDevRef"=w394) -> ("error out"=w401:errorcluster, "RobotDriveDevRef"=w400:T3)  [unwired: 5 in, 1 out]
          n131 = call <vilib>:"WPI_RobotDriveDelayAndUpdateSafety.vi"("error in (no error)"=w401, "Delay (s)"=1.4, "RobotDriveDevRef"=w400) -> ("error out"=w409:errorcluster, "RobotDriveDevRef 2"=w408:T3)  [unwired: 7 in]
          n132 = call-poly <vilib>:"WPI_RobotDriveArcadeDrive.vi"("error in (no error)"=w409, "Y axis value"=0.0, "RobotDriveDevRef"=w408) -> ("error out"=w403:errorcluster, "RobotDriveDevRef"=w406:T3)  [unwired: 6 in, 1 out]
          n133 = call <vilib>:"WPI_MotorControlSetOutput.vi"("error in (no error)"=w403, "Output"=0.0, "MotorControlDevRef"=w393) -> ("error out"=w404:errorcluster)  [unwired: 6 in, 2 out]
          n134 = call <vilib>:"WPI_MotorControlSetOutput.vi"("error in (no error)"=w404, "Output"=0.0, "MotorControlDevRef"=w392) -> ("error out"=w402:errorcluster)  [unwired: 6 in, 2 out]
          n135 = call <vilib>:"WPI_RobotDriveDelayAndUpdateSafety.vi"("error in (no error)"=w402, "Delay (s)"=0.5, "RobotDriveDevRef"=w406) -> ()  [unwired: 7 in, 2 out]
        }
        frame "LLL", "LR", Default {
          n136 = call <vilib>:"WPI_RobotDriveTankDrive.vi"("error in (no error)"=w413, "Right axis value"=0.82 ("Y axis value"), "Left axis value"=0.8 ("X axis value"), "RobotDriveDevRef"=w414) -> ("error out"=w438:errorcluster, "RobotDriveDevRef"=w437:T3)  [unwired: 5 in, 1 out]
          n137 = call <vilib>:"WPI_RobotDriveDelayAndUpdateSafety.vi"("error in (no error)"=w438, "Delay (s)"=1.6, "RobotDriveDevRef"=w437) -> ("error out"=w426:errorcluster, "RobotDriveDevRef 2"=w427:T3)  [unwired: 7 in]
          n138 = call <vilib>:"WPI_RobotDriveTankDrive.vi"("error in (no error)"=w426, "Right axis value"=-0.8 ("Y axis value"), "Left axis value"=0.8 ("X axis value"), "RobotDriveDevRef"=w427) -> ("error out"=w431:errorcluster, "RobotDriveDevRef"=w430:T3)  [unwired: 5 in, 1 out]
          n139 = call <vilib>:"WPI_RobotDriveDelayAndUpdateSafety.vi"("error in (no error)"=w431, "Delay (s)"=0.35, "RobotDriveDevRef"=w430) -> ("error out"=w421:errorcluster, "RobotDriveDevRef 2"=w422:T3)  [unwired: 7 in]
          n140 = call-poly <vilib>:"WPI_RobotDriveArcadeDrive.vi"("error in (no error)"=w421, "Y axis value"=0.8, "RobotDriveDevRef"=w422) -> ("error out"=w417:errorcluster, "RobotDriveDevRef"=w419:T3)  [unwired: 6 in, 1 out]
          n141 = call <vilib>:"WPI_RobotDriveDelayAndUpdateSafety.vi"("error in (no error)"=w417, "Delay (s)"=0.6, "RobotDriveDevRef"=w419) -> ("error out"=w416:errorcluster, "RobotDriveDevRef 2"=w418:T3)  [unwired: 7 in]
          n142 = call-poly <vilib>:"WPI_RobotDriveArcadeDrive.vi"("error in (no error)"=w416, "Y axis value"=0.5, "RobotDriveDevRef"=w418) -> ("error out"=w440:errorcluster, "RobotDriveDevRef"=w443:T3)  [unwired: 6 in, 1 out]
          n143 = call <vilib>:"WPI_MotorControlSetOutput.vi"("error in (no error)"=w440, "Output"=1.0, "MotorControlDevRef"=w412) -> ("error out"=w441:errorcluster)  [unwired: 6 in, 2 out]
          n144 = call <vilib>:"WPI_MotorControlSetOutput.vi"("error in (no error)"=w441, "Output"=-1.0, "MotorControlDevRef"=w411) -> ("error out"=w439:errorcluster)  [unwired: 6 in, 2 out]
          n145 = call <vilib>:"WPI_RobotDriveDelayAndUpdateSafety.vi"("error in (no error)"=w439, "Delay (s)"=0.5, "RobotDriveDevRef"=w443) -> ("error out"=w423:errorcluster, "RobotDriveDevRef 2"=w424:T3)  [unwired: 7 in]
          n146 = call-poly <vilib>:"WPI_RobotDriveArcadeDrive.vi"("error in (no error)"=w423, "Y axis value"=0.0, "RobotDriveDevRef"=w424) -> ()  [unwired: 6 in, 3 out]
        }
      }
    }
  }
